vi "stoperaseDO_tt.vi"   [LabVIEW 2013]
types:
  T1 = typedef "LVRectTypeDef.ctl" = cluster{"Left":i16, "Top":i16, "Right":i16, "Bottom":i16}
  T2 = cluster{"Xpixels":i32, "Vxminref":dbl, "Vxmaxref":dbl, "P":dbl, "Ypixels":i32, "Vyminref":dbl, "Vymaxref":dbl, "srate":sgl, "sAOxy":i32, "timeout":dbl, "type":string, "date":string, "time":string, "Colormap":u16, "Drawing Mode":u16, "Scanning Mode":u16, "square pixels":bool, "square matrix":bool, "Xpixels Img":i32, "Vx-min Img":dbl, "VX-max Img":dbl, "Ypixels Img":i32, "Vy-min Img":dbl, "Vy-max Img ":dbl, "Angle Img":dbl, "autoshutter":bool, "finite":bool, "cont":bool, "wavdet":bool, "measpoints":i32, "avpp":i32, "bufferAO":i32, "bufferAI":i32, "starttick":u32, "waveform":path, "Vx-ref":dbl, "Vy-ref":dbl, "refreshrate":dbl, "refreshbuffer":i32, "tt_cycles":i32, "motorref":refnum<k7>, "mirrorswitch":refnum<k7>, "sample mode":i32, "maxbufferAI":i32, "sampletreshold":dbl, "srateAODO":sgl, "bin":sgl, "Pel":sgl, "Angle draw":dbl, "srate Img":sgl, "ROIimg_plotbounds":T1, "auto OD":bool, "ODfilt":u16, "reset AO_DO":bool, "aAI":i32[], "aCI":i32[], "aAO":i32[], "aDO":i32[]}
  T3 = cluster{"Min Voltage sq (mV)":dbl, "Max voltage sq (mV)":dbl, "Duty cycle sq(%)":dbl, "Voltage freq. sq(Hz)":dbl, "# cycles sq":u32, "meastype":enum16{"sealtest hekcells", "sealtest neurons", "Manual", "from file"}, "sample rate":dbl, "amp":dbl, "sample mode":i32, "refreshbuffer":i32, "timeout":sgl, "Min Voltage tri (mV)":dbl, "Max voltage tri (mV)":dbl, "Voltage freq. tri(Hz)":dbl, "# cycles tri":u32, "Voltage step ":bool, "Voltage triangle":bool, "file":bool, "refreshrate":dbl, "sAOXY":dbl, "avpp":i32, "Pel":dbl, "bin":dbl, "lAO":i32[], "lDO":i32[]}
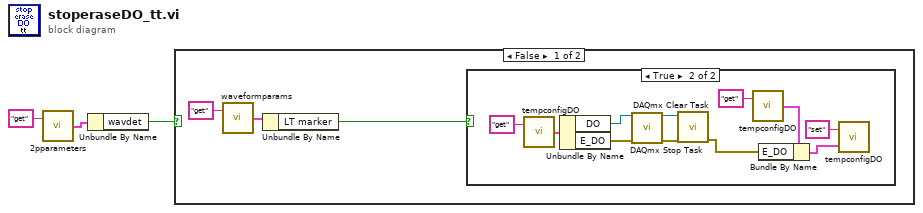
[diagram p0: block diagram]
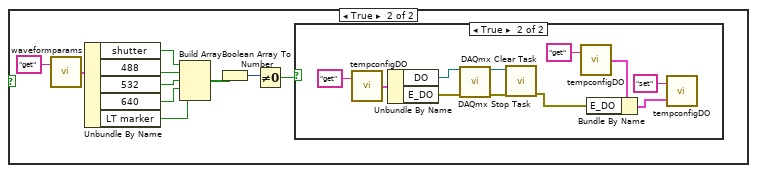
[diagram p3: hidden frame]
diagram:
  n1 = call "2pparameters.vi"("command"="get") -> ("params out"=w2:T2)  [unwired: 1 in]
  n2 = Unbundle By Name(w2) -> ("wavdet"=w1:bool)
  n3 = case shown="False" w1 {
    frame False {
      n4 = call "waveformparams.vi"("command"="get") -> ("Params out"=w5:T3)  [unwired: 1 in]
      n5 = Unbundle By Name(w5) -> ("LT marker"=w4:bool)
      n6 = case shown="True" w4 {
        frame False {
        }
        frame True {
          n7 = call "tempconfigDO.vi"("command"="get") -> ("Temp Config out"=w14:cluster{"DO":refnum<k21>, "E_DO":errorcluster})  [unwired: 1 in]
          n8 = Unbundle By Name(w14) -> ("DO"=w13:refnum<k21>, "E_DO"=w12:errorcluster)
          n9 = call <vilib>:"DAQmx Stop Task.vi"("task/channels in"=w13, "error in"=w12) -> ("task out"=w9:refnum<k21>, "error out"=w8:errorcluster)  [unwired: 12 in]
          n10 = call <vilib>:"DAQmx Clear Task.vi"("task in"=w9, "error in"=w8) -> ("error out"=w7:errorcluster)  [unwired: 13 in]
          n11 = call "tempconfigDO.vi"("command"="get") -> ("Temp Config out"=w11:cluster{"DO":refnum<k21>, "E_DO":errorcluster})  [unwired: 1 in]
          n12 = Bundle By Name(cluster=w11, "E_DO"=w7) -> (w10:cluster{"DO":refnum<k21>, "E_DO":errorcluster})
          n13 = call "tempconfigDO.vi"("Temp Config in"=w10, "command"="set") -> ()  [unwired: 1 out]
        }
      }
    }
    frame True {
      n14 = call "waveformparams.vi"("command"="get") -> ("Params out"=w26:T3)  [unwired: 1 in]
      n15 = Unbundle By Name(w26) -> ("shutter"=w25:bool, "488"=w24:bool, "532"=w23:bool, "640"=w22:bool, "LT marker"=w18:bool)
      n16 = Build Array(w25, w24, w23, w22, w18) -> (w21:bool[])
      n17 = Boolean Array To Number(Boolean array=w21) -> (number=w20:u32)
      n18 = Not Equal To 0?(x=w20) -> (x != 0?=w19:bool)
      n19 = case shown="True" w19 {
        frame False {
        }
        frame True {
          n20 = call "tempconfigDO.vi"("command"="get") -> ("Temp Config out"=w35:cluster{"DO":refnum<k21>, "E_DO":errorcluster})  [unwired: 1 in]
          n21 = Unbundle By Name(w35) -> ("DO"=w34:refnum<k21>, "E_DO"=w33:errorcluster)
          n22 = call <vilib>:"DAQmx Stop Task.vi"("task/channels in"=w34, "error in"=w33) -> ("task out"=w30:refnum<k21>, "error out"=w29:errorcluster)  [unwired: 12 in]
          n23 = call <vilib>:"DAQmx Clear Task.vi"("task in"=w30, "error in"=w29) -> ("error out"=w28:errorcluster)  [unwired: 13 in]
          n24 = call "tempconfigDO.vi"("command"="get") -> ("Temp Config out"=w32:cluster{"DO":refnum<k21>, "E_DO":errorcluster})  [unwired: 1 in]
          n25 = Bundle By Name(cluster=w32, "E_DO"=w28) -> (w31:cluster{"DO":refnum<k21>, "E_DO":errorcluster})
          n26 = call "tempconfigDO.vi"("Temp Config in"=w31, "command"="set") -> ()  [unwired: 1 out]
        }
      }
    }
  }
